vi "Set Static IP.vi"(0 "MAC Address":string, 3 "error in (no error)":errorcluster, 4 "Target Info In":T2) -> (7 "Network Module Information":T1 {"IP Mode" items=["Static"=1, "DHCP/Link-Local"=2, "Link-Local Only"=4, "DHCP Only"=8]}, 10 "error out":errorcluster)   [LabVIEW 2013]
uses:
  types/MAX Sys Cfg Target Information.ctl
  <vilib>/nisyscfg/Initialize (String).vi
  <vilib>/nisyscfg/Save Changes (System).vi
  <vilib>/nisyscfg/Close (System).vi
  <vilib>/nisyscfg/nisyscfg.lvlib
  <resource>/objmgr/nisysapi.rc
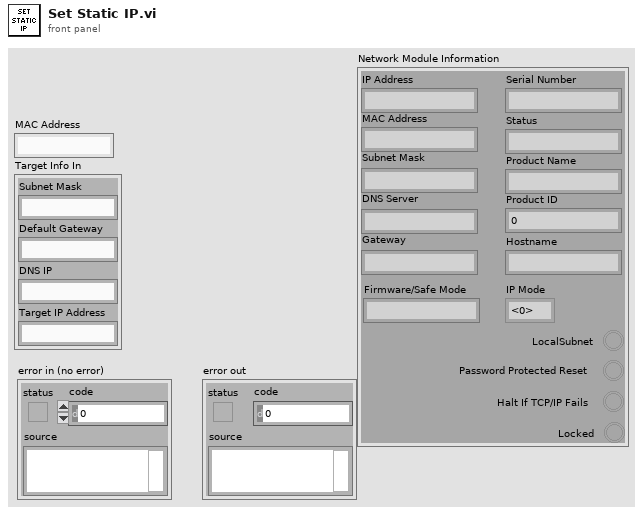
[diagram p1: front panel]
types:
  T1 = typedef "MAX Sys Cfg Target Information.ctl" = cluster{"MAC Address":string, "IP Address":string, "Status":string, "Product Name":string, "Hostname":string, "Firmware/Safe Mode":string, "Subnet Mask":string, "Gateway":string, "DNS Server":string, "Serial Number":string, "Product ID":u32, "Locked ":bool, "LocalSubnet":bool, "Halt If TCP/IP Fails":bool, "Password Protected Reset":bool, "IP Mode":i32}
  T2 = cluster{"Subnet Mask":string, "Default Gateway":string, "DNS IP":string, "Target IP Address":string}
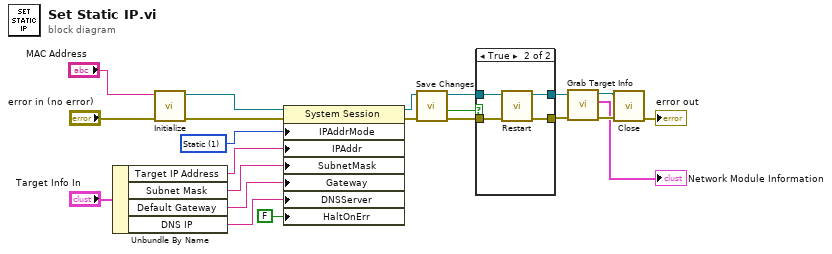
[diagram p0: block diagram]
diagram:
  w21 = 1 items=["Static"=1, "DHCP/Link-Local"=2, "Link-Local Only"=4, "DHCP Only"=8] ("Primary NIC:IP Address Request Mode")
  n1 = Unbundle By Name("Target Info In") -> ("Target IP Address"=w12:string, "Subnet Mask"=w11:string, "Default Gateway"=w10:string, "DNS IP"=w9:string)
  n2 = call-poly <vilib>:"Initialize.vi"("error in (no error)"="error in (no error)", "target (localhost)"="MAC Address") -> ("error out"=w16:errorcluster, "session out"=w15:refnum<k21>)  [unwired: 7 in, 1 out]
  n3 = property class="System Session"(reference=w15, error in=w16, "IPAddrMode"=w21, "IPAddr"=w12, "SubnetMask"=w11, "Gateway"=w10, "DNSServer"=w9, "HaltOnErr"=FALSE ("Real-Time:Halt On IP Error")) -> (reference out=w18:refnum<k21>, error out=w17:errorcluster)
  n4 = call-poly <vilib>:"Save Changes.vi"("error in (no error)"=w17, "session in"=w18) -> ("error out"=w19:errorcluster, "changes require restart"=w6:bool, "session out"=w20:refnum<k21>)  [unwired: 6 in, 1 out]
  n5 = case shown="True" w6 {
    tunnel: [w24 w28] -> w5
    tunnel: [w23 w27] -> w4
    tunnel: w20 -> [w23 w26]
    tunnel: w19 -> [w24 w25]
    frame False {
    }
    frame True {
      n6 = call <vilib>:"Restart.vi"("error in (no error)"=w25, "session in"=w26) -> ("error out"=w28:errorcluster, "session out"=w27:refnum<k21>)  [unwired: 7 in, 1 out]
    }
  }
  n7 = call "Grab Target Info.vi"("error in (no error)"=w5, "Refnum in"=w4) -> ("error out"=w3:errorcluster, "Network Module Information"=→"Network Module Information":T1, "Refnum out"=w2:refnum<k21>)  [unwired: 7 in]
  n8 = call-poly <vilib>:"Close.vi"("error in (no error)"=w3, "session in"=w2) -> ("error out"=→"error out":errorcluster)  [unwired: 9 in]
